vi "Square wave response measurements.vi"() -> ()   [LabVIEW 2021]
uses:
  Waveform generator VIs/Wavegen parameters.ctl
  Waveform generator VIs/Load Impedance.ctl
  Sweep VIs/Log sweep.vi
  Sweep VIs/Linear sweep (linspace).vi
  Waveform generator VIs/Set wavegen SQUare signal parameters.vi
  <instrlib>/Keysight InfiniiVision/Keysight InfiniiVision.lvlib
panel:
  in  "Sweep type":enum16{"Decade", "Linear"}(ring)
  in  "Stop frequency":dbl=26.0 min=0.2
  in  "Start frequency":dbl=25.0 min=0.1 max=20000000.0
  in  "Number of points":i32=2 min=2
  out "ActualPoints":i32
  out "Waveform Graph":dbl[](graph)
  out "Current frequency":dbl
  in  "Offset (V)":dbl format="%#_13g"
  in  "Amplitude (V)":dbl format="%#_13g"
  in  "Simulate":bool=TRUE
  in  "resource string":refnum<visa-resource-name>="USB0::0x0957::0x1798::MY52161667::INSTR" caption="Instrument resource"
  out "error code":i32 caption="Instrument error code" format="%.0g"
  out "Log":string
  out "error message":string caption="Intrument error message"
  in  "NumberOfAverages":i32=500
  # "Waveform generator settings"
  # "Sweep settings"
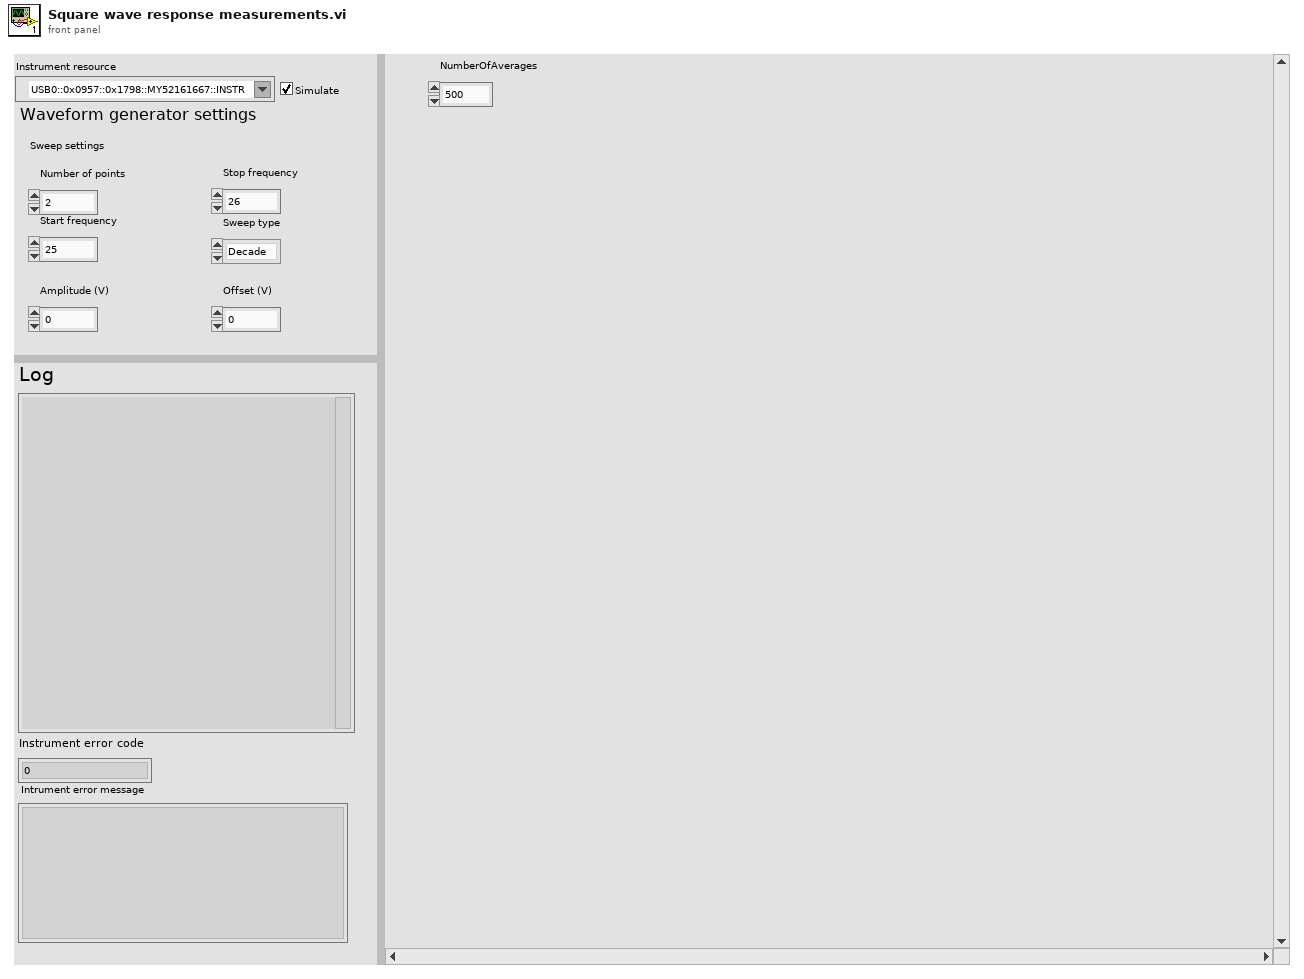
[diagram p1: front panel]
types:
  T1 = typedef "Load Impedance.ctl" = enum16{"ONEMeg", "FIFTy"}
  T2 = typedef "Wavegen parameters.ctl" = cluster{"Frequency (Hz)":dbl, "Amplitude (V)":dbl, "Offset (V)":dbl, "Load Impedance":T1}
  T3 = cluster{"Channel":string, "Preamble":dbl[], "Waveform":dbl[], "Frequency":dbl, "Voltage Pk-Pk":dbl, "Voltage Avg":dbl, "Voltage Min":dbl, "Voltage Max":dbl, "Rise Time":dbl, "Fall Time":dbl, "ActualPoints":i32}
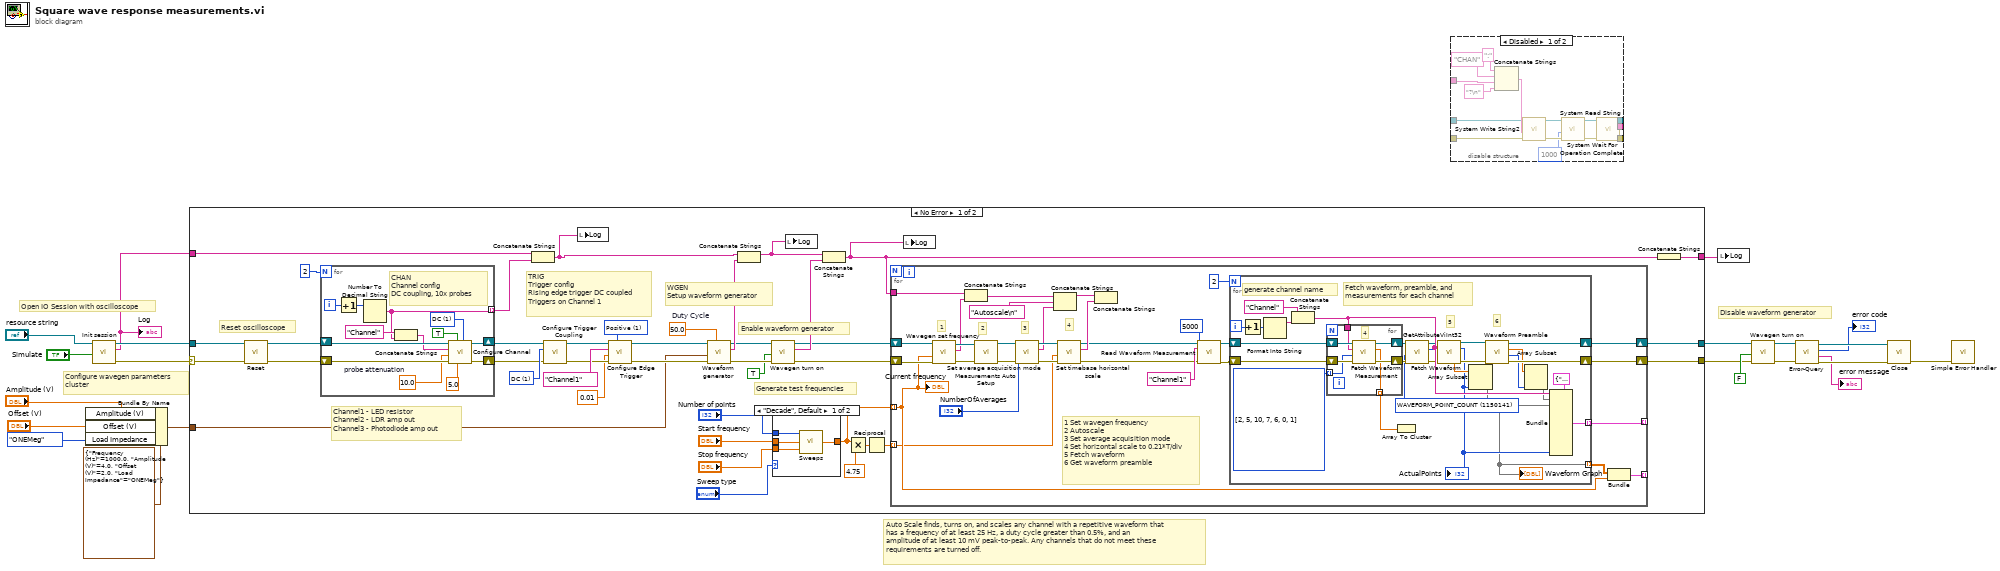
[diagram p0: block diagram]
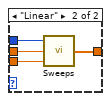
[diagram p2: hidden frame]
diagram:
  # "Auto Scale finds, turns on, and scales any channel with a repetitive waveform that\nhas a frequency of at least 25 Hz, a duty cycle greater than 0.5%, and an\namplitude of at least 10 mV peak-to-peak. Any channels that do not meet these\nrequirements are turned off."
  # "Disable waveform generator"
  # "Configure wavegen parameters\ncluster"
  # "Open IO Session with oscilloscope"
  n1 = Bundle By Name(cluster=T2 {"Frequency (Hz)"=1000.0, "Amplitude (V)"=4.0, "Offset (V)"=2.0, "Load Impedance"=enum."ONEMeg"} ("Wavegen parameters"), "Amplitude (V)"="Amplitude (V)", "Offset (V)"="Offset (V)", "Load Impedance"=Load_Impedance."ONEMeg") -> (w9:T2)
  n2 = call "Init session.vi"("Simulate"="Simulate", "resource string"="resource string") -> ("error out"=w4:errorcluster, "log string out"=w5:string, "instrument handle out"=w16:refnum<k15>)  [unwired: 7 in]
  "Log" <- w5
  n3 = case shown="No Error" w4 {
    selector: w4 -> [w49 w147]
    tunnel: w16 -> [w61 w148]
    tunnel: w5 -> [w50 _]
    tunnel: w9 -> [w31 _]
    tunnel: [w29 _] -> w3
    tunnel: [w24 w148] -> w2
    tunnel: [w23 w147] -> w1
    frame No Error {
      w41 = 50.0  # Duty Cycle
      w54 = 1 items=["Negative", "Positive"] ("trigger slope (Negative)")
      w55 = 1 items=["AC"=0, "DC"=1, "HF Reject"=3, "LF Reject"=4, "Noise Reject"=5] ("trigger coupling (AC)")
      # "Generate test frequencies"
      # "Enable waveform generator"
      # "WGEN\nSetup waveform generator"
      # "TRIG\nTrigger config\nRising edge trigger DC coupled\nTriggers on Channel 1"
      # "Channel1 - LED resistor\nChannel2 - LDR amp out\nChannel3 - Photodiode amp out"
      # "Reset oscilloscope"
      n4 = call <instrlib>:"Reset.vi"("error in (no error)"=w49, "instrument handle"=w61) -> ("error out"=w59:errorcluster, "instrument handle out"=w60:refnum<k15>)  [unwired: 8 in]
      n5 = for {
        N: 2 -> [_]
        shift-right: [w136] -> w48
        shift-left: w60 -> [w146]
        shift-right: [w135] -> w47
        shift-left: w59 -> [w145]
        tunnel: [w137] -> w57 mode=indexing
        i -> [w140]
        w141 = 10.0  # probe attenuation
        w142 = 1 items=["AC", "DC", "Gnd"] ("vertical coupling (AC)")
        # "CHAN\nChannel config\nDC coupling, 10x probes"
        n6 = Increment(x=w140) -> (x+1=w139:i32)
        n7 = Number To Decimal String(number=w139) -> (decimal integer string=w137:string)  [unwired: 1 in]
        n8 = Concatenate Strings("Channel" ("channel name"), w137) -> (w138:string)
        n9 = call <instrlib>:"Configure Channel.vi"("vertical coupling (AC)"=w142, "vertical range"=5.0, "channel enabled (Off)"=TRUE ("channel enabled"), "error in (no error)"=w145, "probe attenuation"=w141, "channel name"=w138, "instrument handle"=w146) -> ("error out"=w135:errorcluster, "instrument handle out"=w136:refnum<k15>)  [unwired: 3 in]
      }
      n10 = Concatenate Strings(w50, w57) -> (w34:string)
      n11 = call <instrlib>:"Configure Trigger Coupling.vi"("error in (no error)"=w47, "trigger coupling (AC)"=w55, "instrument handle"=w48) -> ("error out"=w52:errorcluster, "instrument handle out"=w53:refnum<k15>)  [unwired: 7 in]
      n12 = local write "Log"(w34) -> ()
      n13 = call <instrlib>:"Configure Edge Trigger.vi"("trigger slope (Negative)"=w54, "error in (no error)"=w52, "trigger level"=0.01, "trigger source"="Channel1", "instrument handle"=w53) -> ("error out"=w32:errorcluster, "instrument handle out"=w33:refnum<k15>)  [unwired: 5 in]
      n14 = call-poly "Waveform generator.vi"("Duty Cycle"=w41, "error in (no error)"=w32, "Wavegen parameters in"=w31, "instrument handle in"=w33) -> ("error out"=w42:errorcluster, "log string out"=w45:string, "instrument handle out"=w43:refnum<k15>)  [unwired: 5 in]
      n15 = Concatenate Strings(w34, w45) -> (w46:string)
      n16 = call "Wavegen turn on.vi"("error in (no error)"=w42, "Output Enabled (TRUE)"=TRUE, "IVI Refnum in"=w43) -> ("error out"=w35:errorcluster, "log string out"=w44:string, "IVI Refnum out"=w36:refnum<k15>)  [unwired: 6 in]
      n17 = case shown="\"Decade\", Default" "Sweep type" {
        tunnel: "Stop frequency" -> [w63 w69]
        tunnel: "Start frequency" -> [w64 w68]
        tunnel: "Number of points" -> [w65 w67]
        tunnel: [w62 w66] -> w25
        frame "Decade", Default {
          n18 = call-poly "Sweeps.vi"("Stop frequency"=w63, "Start frequency"=w64, "Number of points"=w65) -> ("log10 space out"=w62:dbl[])
        }
        frame "Linear" {
          n19 = call-poly "Sweeps.vi"("Stop frequency"=w69, "Start frequency"=w68, "Number of points"=w67) -> ("linspace"=w66:dbl[])
        }
      }
      n20 = local write "Log"(w46) -> ()
      n21 = Concatenate Strings(w46, w44) -> (w22:string)
      n22 = Multiply(x=w25, y=4.75) -> (x*y=w26:dbl[])
      n23 = Reciprocal(x=w26) -> (1/x=w27:dbl[])
      n24 = for {
        shift-right: [w79] -> w24
        shift-left: w36 -> [w87]
        shift-right: [w78] -> w23
        shift-left: w35 -> [w86]
        tunnel: w27 -> [w77] mode=indexing
        tunnel: [w98] -> _ mode=indexing
        tunnel: [w88] -> _ mode=indexing
        tunnel: w25 -> [w83] mode=indexing
        tunnel: w22 -> [w82]
        # "4"
        # "3"
        # "1 Set wavegen frequency\n2 Autoscale\n3 Set average acquisition mode\n4 Set horizontal scale to 0.21*T/div\n5 Fetch waveform\n6 Get waveform preamble"
        # "2"
        # "1"
        n25 = call "Wavegen set frequency.vi"("error in (no error)"=w86, "Frequency (Hz)"=w83, "IVI Refnum in"=w87) -> ("error out"=w84:errorcluster, "log string out"=w81:string, "IVI Refnum out"=w85:refnum<k15>)  [unwired: 6 in]
        n26 = Concatenate Strings(w82, w81) -> (w76:string)
        n27 = call <instrlib>:"Measurements Auto Setup.vi"("error in (no error)"=w84, "instrument handle"=w85) -> ("error out"=w96:errorcluster, "instrument handle out"=w97:refnum<k15>)  [unwired: 8 in]
        n28 = call "Set average acquisition mode.vi"("error in (no error)"=w96, "NumberOfAverages"="NumberOfAverages", "IVI Refnum in"=w97) -> ("error out"=w94:errorcluster, "log string out"=w74:string, "IVI Refnum out"=w95:refnum<k15>)  [unwired: 6 in]
        n29 = Concatenate Strings(w76, "Autoscale\n" ("string"), w74) -> (w72:string)
        n30 = call "Set timebase horizontal scale.vi"("error in (no error)"=w94, "Horizontal timebase scale"=w77, "IVI Refnum in"=w95) -> ("error out"=w70:errorcluster, "log string out"=w73:string, "IVI Refnum out"=w71:refnum<k15>)  [unwired: 6 in]
        n31 = Concatenate Strings(w72, w73) -> ()  [unwired: 1 out]
        n32 = call <instrlib>:"Read Waveform Measurement.vi"("instrument handle"=w71, "channel name"="Channel1", "maximum time"=5000, "error in (no error)"=w70) -> ("instrument handle out"=w93:refnum<k15>, "error out"=w92:errorcluster)  [unwired: 9 in, 1 out]
        n33 = for {
          N: 2 -> [_]
          shift-right: [w107] -> w79
          shift-left: w93 -> [w124]
          shift-right: [w113] -> w78
          shift-left: w92 -> [w123]
          tunnel: [w121] -> w98 mode=indexing
          tunnel: [w100] -> w89 mode=indexing
          i -> [w126]
          w101 = u32 1150141 items=["AC_LINE_TRIGGER_SLOPE"=1250701, "ACQUISITION_SEGMENTEDMEMORY_INDEX"=1150139, "ACQUISITION_SEGMENTEDMEMORY_SEGMENT_COUNT"=1150138, "ACQUISITION_TYPE"=1250101, "CHANNEL_COUNT"=1050203, "CHANNEL_PROTECTION"=1150202, "CHANNEL_UNITS"=1150033, "DIGITALCHANNEL_COUNT"=1150038, "DIGITALCHANNEL_POSITION"=1150041, "DIGITALCHANNEL_SIZE"=1150042, "DVM_MODE"=1150443, "EXTERNAL_UNITS"=1150014, "GLITCH_CONDITION"=1250403, "GLITCH_POLARITY"=1250402, "HORZ_MIN_NUM_PTS"=1250009, "HORZ_RECORD_LENGTH"=1250008, "INTERPOLATION"=1250019, "NUM_AVERAGES"=1250104, "NUM_ENVELOPES"=1250105, "REFERENCE_SIGNAL"=1150433, "RUNT_POLARITY"=1250303, "SAMPLE_MODE"=1250106, "STATISTICS_FORMAT"=1150355, "STATUS_SERIAL_POLL"=1150019, "SYSTEM_IO_TIMEOUT"=1150607, "SYSTEM_PRECISION_RECORD_LENGTH"=1150589, "SYSTEM_TIMEOUT_MILLISECONDS"=1150023, "TIMEBASE_MODE"=1150107, "TIMEBASE_TIME_REFERENCE"=1150110, "TRIGGER_ACLINE_SLOPE"=1150556, "TRIGGER_COUPLING"=1250014, "TRIGGER_DELAY_ARMING_SLOPE"=1150263, "TRIGGER_DELAY_EDGE_COUNT"=1150267, "TRIGGER_DELAY_SLOPE"=1150266, "TRIGGER_EDGE_BURST_NTH_EDGE"=1150247, "TRIGGER_EDGE_BURST_SLOPE"=1150249, "TRIGGER_EDGE_REJECT_FILTER_TYPE"=1150135, "TRIGGER_MODIFIER"=1250102, "TRIGGER_PATTERN_CONDITION"=1150195, "TRIGGER_RUNT_CONDITION"=1150189, "TRIGGER_SETUP_AND_HOLD_SLOPE"=1150250, "TRIGGER_SLOPE"=1250018, "TRIGGER_TRANSITION_CONDITION"=1150255, "TRIGGER_TRANSITION_SLOPE"=1150256, "TRIGGER_TYPE"=1250012, "TRIGGER_TYPE_AG"=1150557, "TRIGGER_WIDTH_CONDITION"=1150197, "TRIGGER_WIDTH_POLARITY"=1150200, "VERTICAL_COUPLING"=1250003, "WAVEFORM_BYTE_ORDER"=1150085, "WAVEFORM_DATA_FORMAT"=1150086, "WAVEFORM_POINT_COUNT"=1150141, "WAVEFORM_POINT_MODE"=1150087, "WAVEFORM_SUB_SOOURCE"=1150609, "WAVEFORM_X_REFERENCE"=1150145, "WAVEFORM_Y_REFERENCE"=1150146, "WIDTH_CONDITION"=1250504, "WIDTH_POLARITY"=1250503] ("AttributeID")
          w122 = i32[] [2, 5, 10, 7, 6, 0, 1] items=["Rise Time"=0, "Fall Time"=1, "Frequency"=2, "Period"=3, "Voltage Rms"=4, "Voltage Peak To Peak"=5, "Voltage Max"=6, "Voltage Min"=7, "Voltage High"=8, "Voltage Low"=9, "Voltage Average"=10, "Width Neg"=11, "Width Pos"=12, "Duty Cycle Neg"=13, "Duty Cycle Pos"=14, "Amplitude"=15, "Voltage Cycle Rms"=16, "Voltage Cycle Average"=17, "Overshoot"=18, "Preshoot"=19, "Measurement Time At Max"=21, "Measurement Frequency Counter"=20, "Measurement Time At Min"=22, "Measurement Delay"=23, "Measurement Value At Time"=25, "Measurement Phase"=24, "Measurement Time At Value"=26, "Measurement Time Of Edge"=27, "Measurement Area"=28, "Measurement Burst Width"=29, "Measurement Falling Edge Count"=30, "Measurement Rising Edge Count"=32, "Measurement Falling Pulse Count"=31, "Measurement Rising Pulse Count"=33, "Measurement Standard Deviation"=34] ("MeasFunction (Rise Time)")
          # "generate channel name"
          # "6"
          # "Fetch waveform, preamble, and \nmeasurements for each channel"
          # "5"
          n34 = Increment(x=w126) -> (x+1=w125:i32)
          n35 = Format Into String(w125) -> (resulting string=w120:string)  [unwired: 3 in, 1 out]
          n36 = Concatenate Strings("Channel" ("string"), w120) -> (w118:string)
          n37 = for {
            tunnel: w122 -> [w128] mode=indexing
            shift-right: [w130] -> w103
            shift-left: w124 -> [w133]
            shift-right: [w129] -> w102
            shift-left: w123 -> [w132]
            tunnel: w118 -> [w131]
            tunnel: [w127] -> w117 mode=indexing
            # "4"
            n38 = call <instrlib>:"Fetch Waveform Measurement.vi"("error in (no error)"=w132, "measurement function (Rise Time)"=w128, "channel name"=w131, "instrument handle"=w133) -> ("error out"=w129:errorcluster, "measurement"=w127:dbl, "instrument handle out"=w130:refnum<k15>)  [unwired: 5 in]
          }
          n39 = Array To Cluster(array=w117) -> ()  [unwired: 1 out]
          n40 = call <instrlib>:"GetAttributeViInt32.vi"("error in (no error)"=w102, "AttributeID"=w101, "instrument handle"=w103) -> ("error out"=w106:errorcluster, "AttributeValue"=w105:i32, "instrument handle out"=w104:refnum<k15>)  [unwired: 6 in]
          n41 = call <instrlib>:"Fetch Waveform.vi"("instrument handle"=w104, "channel name"=w118, "waveform size (2048)"=w105, "error in (no error)"=w106) -> ("instrument handle out"=w115:refnum<k15>, "actual points"=w108:i32, "waveform array (V)"=w116:dbl[], "error out"=w114:errorcluster)  [unwired: 6 in, 2 out]
          "ActualPoints" <- w108
          n42 = Array Subset(array=w116, length=w108) -> (w100:dbl[])  [unwired: 1 in]
          "Waveform Graph" <- w100
          n43 = call <instrlib>:"Waveform Preamble.vi"("error in (no error)"=w114, "instrument handle"=w115) -> ("error out"=w113:errorcluster, "ValActualSize"=w111:i32, "Val"=w112:dbl[], "instrument handle out"=w107:refnum<k15>)  [unwired: 6 in]
          n44 = Array Subset(array=w112, length=w111) -> (w110:dbl[])  [unwired: 1 in]
          n45 = Bundle(cluster=T3 {"Channel"="", "Preamble"=[], "Waveform"=[], "Frequency"=0.0, "Voltage Pk-Pk"=0.0, "Voltage Avg"=0.0, "Voltage Min"=0.0, "Voltage Max"=0.0, "Rise Time"=0.0, "Fall Time"=0.0, "ActualPoints"=0}, "Channel"=w118, "Preamble"=w110, "Waveform"=w100, "ActualPoints"=w108) -> (w121:T3)  [unwired: 7 in]
        }
        n46 = Bundle(w89, w83) -> (w88:cluster{dbl[][], dbl})  [unwired: 1 in]
        "Current frequency" <- w83
      }
      n47 = local write "Log"(w22) -> ()
      n48 = Concatenate Strings(w22) -> (w29:string)
    }
    frame Error {
    }
  }
  n49 = disable-structure shown="Disabled" {
    disable-tunnel: [w156 _] -> _
    disable-tunnel: [w155 _] -> _
    disable-tunnel: [w154 _] -> _
    disable-tunnel: _ -> [w151 _]
    disable-tunnel: _ -> [w150 _]
    disable-tunnel: _ -> [w149 _]
    frame Disabled {
      n50 = Concatenate Strings(":" ("string"), "CHAN" ("string"), w151, "?\n" ("string")) -> (w162:string)
      n51 = call <instrlib>:"System Write String2.vi"("error in (no error)"=w149, "Data"=w162, "instrument handle"=w150) -> ("error out"=w161:errorcluster, "instrument handle out"=w160:refnum<k15>)  [unwired: 7 in]
      n52 = call <instrlib>:"System Wait For Operation Complete.vi"("error in (no error)"=w161, "MaxTimeMilliseconds"=1000, "instrument handle"=w160) -> ("error out"=w158:errorcluster, "instrument handle out"=w157:refnum<k15>)  [unwired: 7 in]
      n53 = call <instrlib>:"System Read String.vi"("error in (no error)"=w158, "instrument handle"=w157) -> ("error out"=w155:errorcluster, "Val"=w154:string, "instrument handle out"=w156:refnum<k15>)  [unwired: 7 in]
    }
    frame Enabled {
    }
  }
  n54 = local write "Log"(w3) -> ()
  n55 = call "Wavegen turn on.vi"("error in (no error)"=w1, "Output Enabled (TRUE)"=FALSE, "IVI Refnum in"=w2) -> ("error out"=w6:errorcluster, "IVI Refnum out"=w7:refnum<k15>)  [unwired: 6 in, 1 out]
  n56 = call <instrlib>:"Error-Query.vi"("error in (no error)"=w6, "instrument handle"=w7) -> ("error out"=w19:errorcluster, "error message"=→"error message":string, "error code"=→"error code":i32, "instrument handle out"=w20:refnum<k15>)  [unwired: 6 in]
  n57 = call <instrlib>:"Close.vi"("error in (no error)"=w19, "instrument handle"=w20) -> ("error out"=w21:errorcluster)  [unwired: 9 in]
  n58 = call <vilib>:"Simple Error Handler.vi"("error in (no error)"=w21) -> ()  [unwired: 4 in, 5 out]
